vi "DataTree_LS1.vi"(0 "Arbre":refnum<vi>, 1 "Data Folder Path":path, 2 "ScanParamsIn":T1[](array[typedef]), 3 "VarParam":string, 5 "Date String":string="All" caption="Date String (yymmdd)", 9 "Session":i32=-1, 11 "error in (no error)":errorcluster, 12 "IncludeSubF":bool, 13 "Recheck Files":bool, 14 "KeyWord":string) -> (4 "Arbre Out":refnum<vi>, 6 "Headers":T1[](array[typedef]), 10 "Tous les tags":string[](array[string]), 15 "error out":errorcluster)   [LabVIEW 2012]
uses:
  Interface Class/ScanParams.ctl
  Interface Class/Interface.lvclass
panel:
  out "Tag Courbes":string[](array[string])
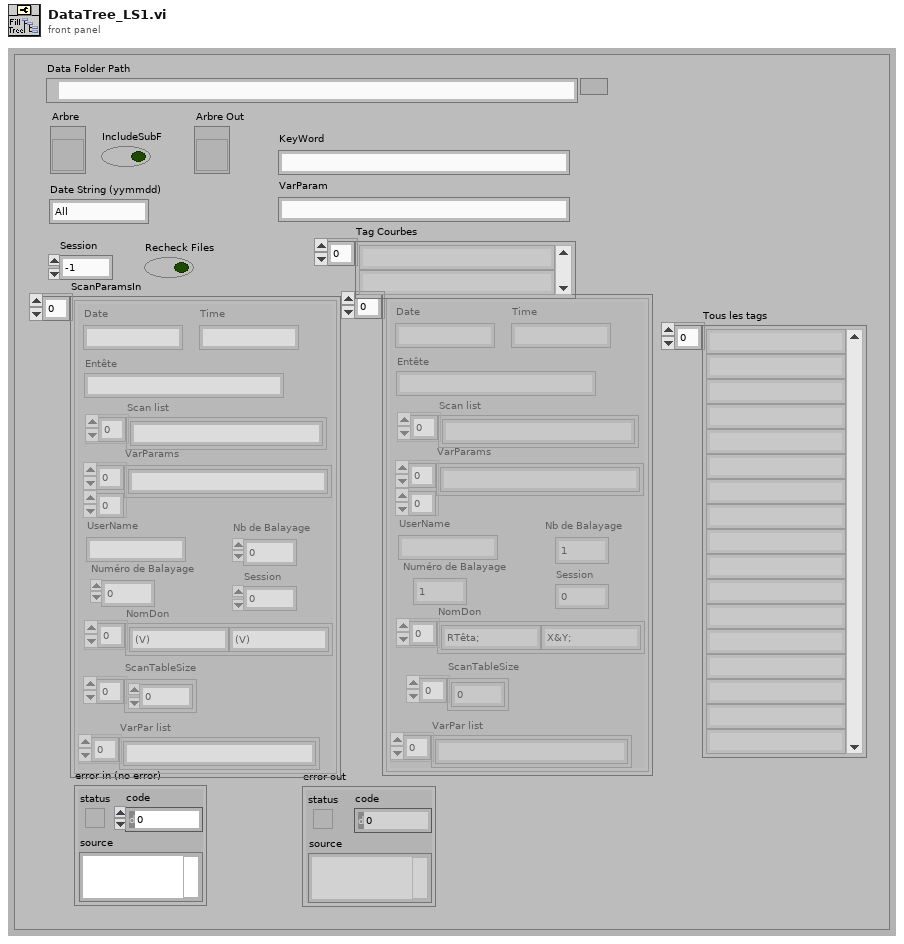
[diagram p1: front panel]
types:
  T1 = typedef "Interface.lvclass/ScanParams.ctl" = cluster{"Entête":string, "Scan list":string[], "NbCourbe":i32, "IndCourbe":i64, "NomDon":string[], "Session ":i32, "Date":string, "Time":string, "VarParams":string[][], "UserName":string, "ScanTableSize":i32[], "VarPar list":string[]}
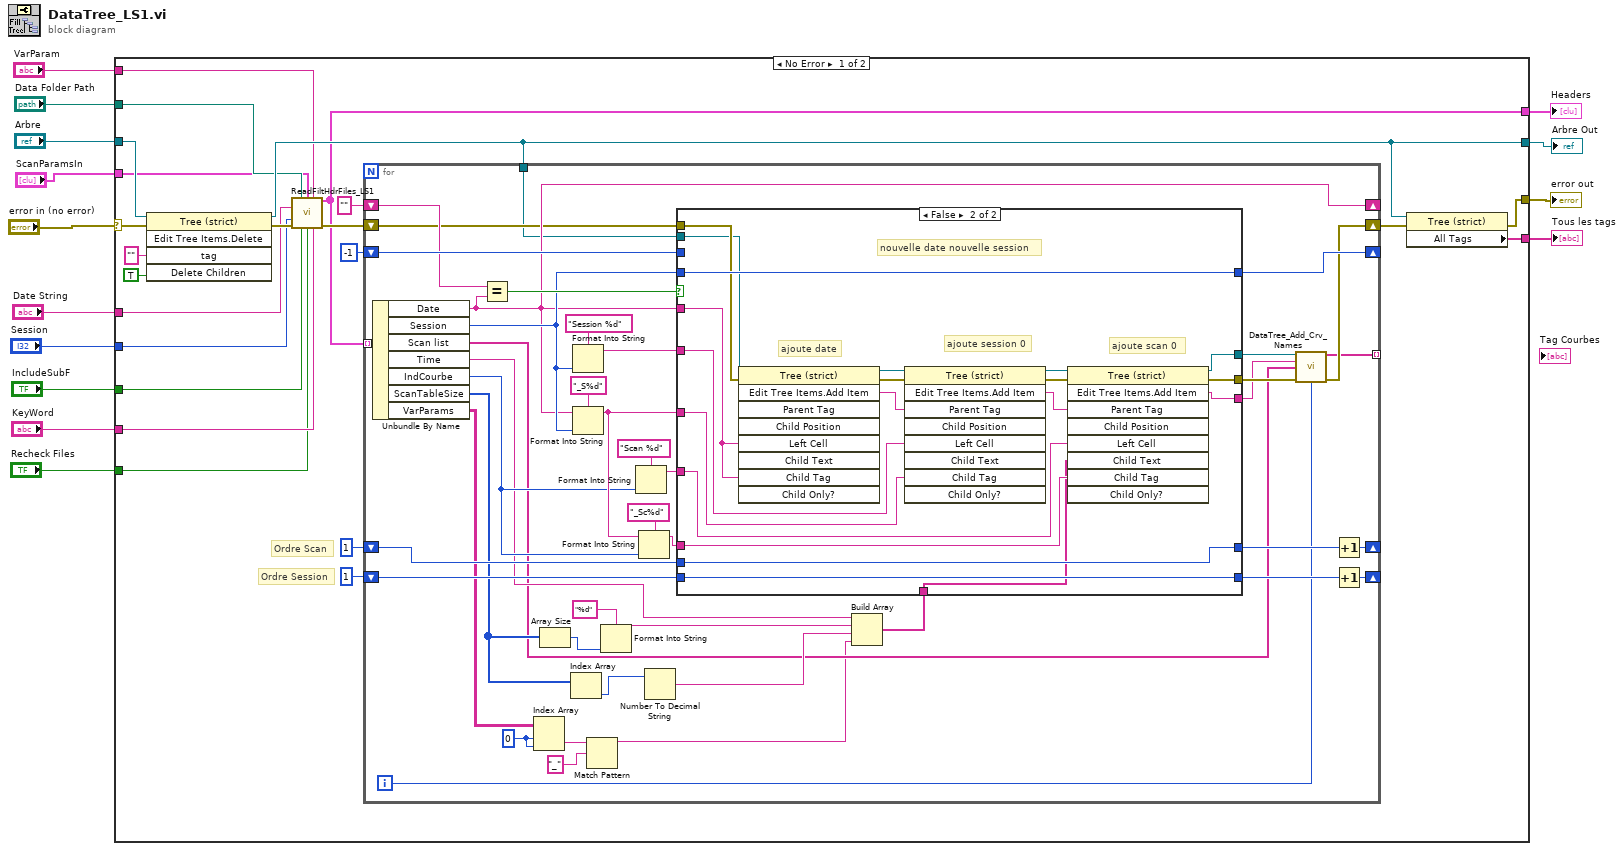
[diagram p0: block diagram]
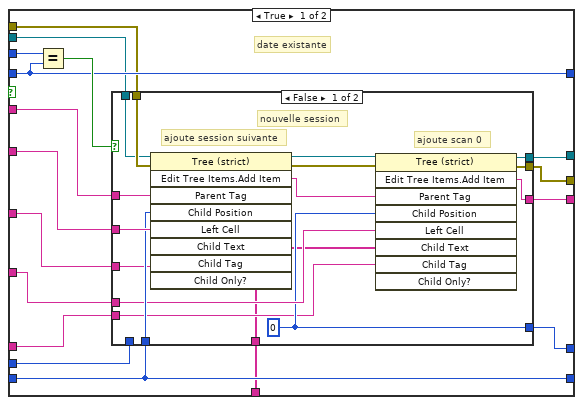
[diagram p2: hidden frame]
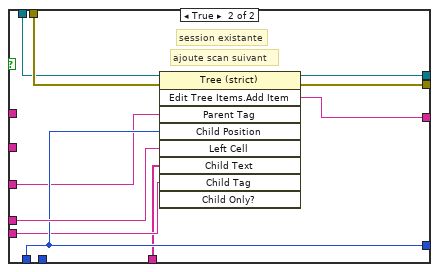
[diagram p3: hidden frame]
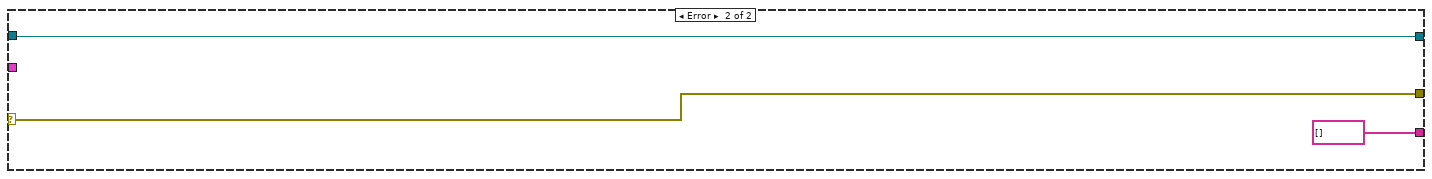
[diagram p4: hidden frame]
diagram:
  n1 = case shown="No Error" "error in (no error)" {
    selector: "error in (no error)" -> [w28 w147]
    tunnel: [w37 string[] [] ("All Tags")] -> w14
    tunnel: [w30 w147] -> w12
    tunnel: [w20 _] -> w11
    tunnel: "Arbre" -> [w25 w145]
    tunnel: [w24 w145] -> w9
    tunnel: "Date String" -> [w23 _]
    tunnel: "Session" -> [w22 _]
    tunnel: "Data Folder Path" -> [w21 _]
    tunnel: "IncludeSubF" -> [w19 _]
    tunnel: "KeyWord" -> [w18 _]
    tunnel: "VarParam" -> [w17 _]
    tunnel: "ScanParamsIn" -> [w16 _]
    tunnel: "Recheck Files" -> [w15 _]
    frame No Error {
      # "Ordre Scan"
      # "Ordre Session"
      n2 = invoke on="Nœud de méthode" class="Tree (strict)" method="Edit Tree Items.Delete"(reference=w25, error in=w28, "tag"="" ("Tag"), "Delete Children"=TRUE ("Supprimer les enfants ?")) -> (reference out=w24:refnum<vi>, error out=w27:errorcluster)  [unwired: 1 in, 3 out]
      n3 = call "ReadFiltHdrFiles_LS1.vi"("Data Folder Path"=w21, "ScanParamsIn"=w16, "VarParam"=w17, "Date String"=w23, "Session"=w22, "error in (no error)"=w27, "IncludeSubF"=w19, "Recheck Files"=w15, "KeyWord"=w18) -> ("ScanParamsOut"=w20:T1[], "error out"=w31:errorcluster)  [unwired: 5 in]
      n4 = for {
        tunnel: w20 -> [w81] mode=indexing
        shift-right: [w64] -> _
        shift-left: "" ("Date") -> [w72]
        shift-right: [w79] -> _
        shift-left: -1 ("Session") -> [w78]
        shift-right: [w77] -> _
        shift-left: 1 ("Session") -> [w73]
        shift-right: [w74] -> _
        shift-left: 1 ("Position de l'enfant") -> [w76]
        shift-right: [w59] -> w32
        shift-left: w31 -> [w61]
        tunnel: w24 -> [w55]
        tunnel: [w54] -> _ mode=indexing
        i -> [w44]
        w40 = 0 ("indice (ligne)")
        n5 = Unbundle By Name(w81) -> ("Date"=w64:string, "Session"=w65:i32, "Scan list"=w43:string[], "Time"=w48:string, "IndCourbe"=w52:i64, "ScanTableSize"=w51:i32[], "VarParams"=w39:string[][])
        n6 = Equal?(x=w72, y=w64) -> (x = y?=w80:bool)
        n7 = Index Array(array=w39, index (row)=w40, index (col)=w40) -> (element=w42:string)
        n8 = Array Size(array=w51) -> (size(s)=w50:i32)
        n9 = Index Array(array=w51) -> (element=w53:i32)  [unwired: 1 in]
        n10 = Format Into String(format string="Session %d" ("chaîne de format"), w65) -> (resulting string=w62:string)  [unwired: 2 in, 1 out]
        n11 = Format Into String(format string="_S%d" ("chaîne de format"), initial string=w64, w65) -> (resulting string=w63:string)  [unwired: 1 in, 1 out]
        n12 = Match Pattern(string=w42, regular expression="_" ("expression régulière")) -> (before substring=w38:string)  [unwired: 1 in, 3 out]
        n13 = Format Into String(format string="%d" ("chaîne de format"), w50) -> (resulting string=w47:string)  [unwired: 2 in, 1 out]
        n14 = Format Into String(format string="Scan %d" ("chaîne de format"), w52) -> (resulting string=w69:string)  [unwired: 2 in, 1 out]
        n15 = Format Into String(format string="_Sc%d" ("chaîne de format"), initial string=w63, w52) -> (resulting string=w68:string)  [unwired: 1 in, 1 out]
        n16 = Number To Decimal String(number=w53) -> (decimal integer string=w46:string)  [unwired: 1 in]
        n17 = Build Array(w48, w47, w46, w38) -> (w45:string[])
        n18 = case shown="False" w80 {
          tunnel: w64 -> [w95 w142]
          tunnel: w65 -> [w88 w143]
          tunnel: [w88 w143] -> w79
          tunnel: w78 -> [w89 _]
          tunnel: w73 -> [w97 w131]
          tunnel: [w96 w131] -> w60
          tunnel: w76 -> [w94 w141]
          tunnel: [w94 w141] -> w75
          tunnel: w69 -> [w93 w137]
          tunnel: w68 -> [w92 w130]
          tunnel: w63 -> [w91 w135]
          tunnel: w62 -> [w90 w136]
          tunnel: w61 -> [w86 w134]
          tunnel: [w87 w133] -> w57
          tunnel: [w85 w132] -> w58
          tunnel: w55 -> [w84 w129]
          tunnel: [w83 w126] -> w56
          tunnel: w45 -> [w82 w125]
          frame True {
            # "date existante"
            n19 = Equal?(x=w89, y=w88) -> (x = y?=w98:bool)
            n20 = case shown="False" w98 {
              tunnel: w90 -> [w113 _]
              tunnel: w95 -> [w114 _]
              tunnel: w97 -> [_ w123]
              tunnel: [w108 w123] -> w96
              tunnel: w94 -> [w112 _]
              tunnel: [w106 w119] -> w85
              tunnel: w91 -> [w107 w122]
              tunnel: w93 -> [w109 w124]
              tunnel: w92 -> [w103 w121]
              tunnel: [w105 w120] -> w87
              tunnel: w86 -> [w104 w118]
              tunnel: w84 -> [w102 w117]
              tunnel: [w100 w116] -> w83
              tunnel: w82 -> [w99 w115]
              frame False {
                w108 = 0 ("Session")
                # "ajoute scan 0"
                # "ajoute session suivante"
                # "nouvelle session"
                n21 = invoke on="Nœud de méthode" class="Tree (strict)" method="Edit Tree Items.Add Item"(reference=w102, error in=w104, "Parent Tag"=w114, "Child Position"=w112, "Left Cell"=w113, "Child Tag"=w107) -> (reference out=w101:refnum<vi>, error out=w111:errorcluster, "Edit Tree Items:Add Item"=w110:string)  [unwired: 3 in, 6 out]
                n22 = invoke on="Nœud de méthode" class="Tree (strict)" method="Edit Tree Items.Add Item"(reference=w101, error in=w111, "Parent Tag"=w110, "Child Position"=w108, "Left Cell"=w109, "Child Text"=w99, "Child Tag"=w103) -> (reference out=w100:refnum<vi>, error out=w106:errorcluster, "Edit Tree Items:Add Item"=w105:string)  [unwired: 2 in, 6 out]
              }
              frame True {
                # "ajoute scan suivant"
                # "session existante"
                n23 = invoke on="Nœud de méthode" class="Tree (strict)" method="Edit Tree Items.Add Item"(reference=w117, error in=w118, "Parent Tag"=w122, "Child Position"=w123, "Left Cell"=w124, "Child Text"=w115, "Child Tag"=w121) -> (reference out=w116:refnum<vi>, error out=w119:errorcluster, "Edit Tree Items:Add Item"=w120:string)  [unwired: 2 in, 6 out]
              }
            }
          }
          frame False {
            # "ajoute date"
            # "ajoute scan 0"
            # "ajoute session 0"
            # "nouvelle date nouvelle session"
            n24 = invoke on="Nœud de méthode" class="Tree (strict)" method="Edit Tree Items.Add Item"(reference=w129, error in=w134, "Left Cell"=w142, "Child Tag"=w142) -> (reference out=w128:refnum<vi>, error out=w144:errorcluster, "Edit Tree Items:Add Item"=w138:string)  [unwired: 5 in, 6 out]
            n25 = invoke on="Nœud de méthode" class="Tree (strict)" method="Edit Tree Items.Add Item"(reference=w128, error in=w144, "Parent Tag"=w138, "Left Cell"=w136, "Child Tag"=w135) -> (reference out=w127:refnum<vi>, error out=w140:errorcluster, "Edit Tree Items:Add Item"=w139:string)  [unwired: 4 in, 6 out]
            n26 = invoke on="Nœud de méthode" class="Tree (strict)" method="Edit Tree Items.Add Item"(reference=w127, error in=w140, "Parent Tag"=w139, "Left Cell"=w137, "Child Text"=w125, "Child Tag"=w130) -> (reference out=w126:refnum<vi>, error out=w132:errorcluster, "Edit Tree Items:Add Item"=w133:string)  [unwired: 3 in, 6 out]
          }
        }
        n27 = call "DataTree_Add_Crv_Names.vi"("référence"=w56, "Parent Name"=w57, "Scan list"=w43, "Entrée d'erreur"=w58, "FileIndex"=w44) -> ("Tag Courbes"=w54:string[], "Sortie d'erreur"=w59:errorcluster)  [unwired: 9 in]
        n28 = Increment(x=w60) -> (x+1=w77:i32)
        n29 = Increment(x=w75) -> (x+1=w74:i32)
      }
      n30 = property on="Nœud de propriété" class="Tree (strict)"(reference=w24, error in=w32) -> (error out=w30:errorcluster, "All Tags"=w37:string[])  [unwired: 1 out]
    }
    frame Error {
    }
  }
  "Tous les tags" <- w14
  "error out" <- w12
  "Headers" <- w11
  "Arbre Out" <- w9
